vi "Init.vi"(6 "Column Definitions":T9[](array[typedef]) {"MinWidth" min=2 step=1; "AutoSizeMode" items=["None"=1, "ColumnHeader"=2, "AllCellsExceptHeader"=4, "AllCells"=6, "DisplayedCellsExceptHeader"=8, "DisplayedCells"=10, "Fill"=16]; "FillWeight" min=1 max=100}, 7 "Menu Items":string[](array[string])=["Add", "Remove", "Edit"], 8 "error in (no error)":errorcluster, 9 "Node object refs":T1, 10 "Event References":T2, 11 "Multi Column Listbox in":refnum<class "Multi Column Listbox.lvclass">) -> (0 "error out":errorcluster, 2 "Table Events":T13, 3 "Multi Column Listbox out":refnum<class "Multi Column Listbox.lvclass">)   [LabVIEW 2013, in "Table Manager.lvlib" / "Multi Column Listbox.lvclass"]
doc: "This VIs creates the Column Objects that the table will use based on the configuration recived, and register the events the table will use. Also creates the evetns that will be used by the table"
uses:
  Multi Column Listbox.lvclass
  Table Manager/Table Events.ctl
  Table Manager/Menu Select.ctl
  Column/Column Descriptor.ctl
  Column/Column.lvclass
  Column/Column Type.ctl
  <vilib>/NI/Tag Bus/tag/Data Type.ctl
  Table Manager/Call Back Ref Type Def.ctl
  Configuration Editor/Classes/Engine Parent/Engine Parent Editor Node.lvclass
  Configuration Editor/Classes/Module editor node/module editor node.lvclass
  Table Manager/references.ctl
  <vilib>/NI/Configuration Framework/Node/StopEvent.ctl
  <vilib>/NI/Configuration Framework/Node/RefreshUIEvent.ctl
  <vilib>/NI/Configuration Framework/Node/CacheState.ctl
  <vilib>/NI/Configuration Framework/Node/NodeChangeEvent.ctl
  <vilib>/NI/Configuration Framework/Node/NodeRef.ctl
  <vilib>/NI/Configuration Framework/Node/NISE_CEF_Node.lvclass
  control module/editor node/channel action event.ctl
  control module/editor node/dialog output action.ctl
  <vilib>/NI/Tag Bus Module Framework/channel/TBM channel.lvclass
  <vilib>/NI/Tag Bus/tag/tag descriptor.lvclass
  <vilib>/NI/AMC/Message Queue.ctl
  <vilib>/NI/AMC/Message.ctl
  <vilib>/NI/Tools/Keyed Array/KeyedArray.ctl
  <vilib>/NI/Configuration Framework/Node/UserEventRef.ctl
  <vilib>/NI/Configuration Framework/Controls/EventCluster.ctl
  Table Manager/object ref.ctl
  Line/Line.lvclass
  Table Manager/Table Manager.lvclass/Table Manager.ctl
  Multi Column Listbox.lvclass/Multi Column Listbox.ctl
  String Column/String Column.lvclass
  Column/Column.lvclass/Column.ctl
  Listbox Enum Column/List Box Enum Column.lvclass
  Listbox Enum Column/List Box Enum Column.lvclass/List Box Enum Column.ctl
  Mapping Column/Mapping Column.lvclass
  Mapping Column/Mapping Column.lvclass/Mapping Column.ctl
  Line/Line.lvclass/Line.ctl
  Column/Write Header.vi
  Column/Write Read Only.vi
  Column/Write Call Back VI.vi
  Listbox Enum Column/Write Enum Reference.vi
  Mapping Column/Write Channel suffix.vi
  Column/Write Dependencies List.vi
  Mapping Column/Write Data Type Dependecy.vi
  Mapping Column/Write Name Dependecy.vi
  Table Manager/Write ATM.vi
  Read Listbox.vi
  Line/Write Line UID.vi
  Line/Write Columns.vi
  Table Manager/Write Line.vi
  Table Manager/Write Menu Selection.vi
  Table Manager/Write object refs.vi
  control module/editor node/control module editor.lvclass
  Table Manager/Table Manager.lvclass
  <vilib>/NI/Tools/Keyed Array/Tools_KeyedArray.lvlib
  <vilib>/NI/AMC/AMC.lvlib
  <vilib>/NI/Configuration Framework/NISE_CEF_TreeControl.lvlib
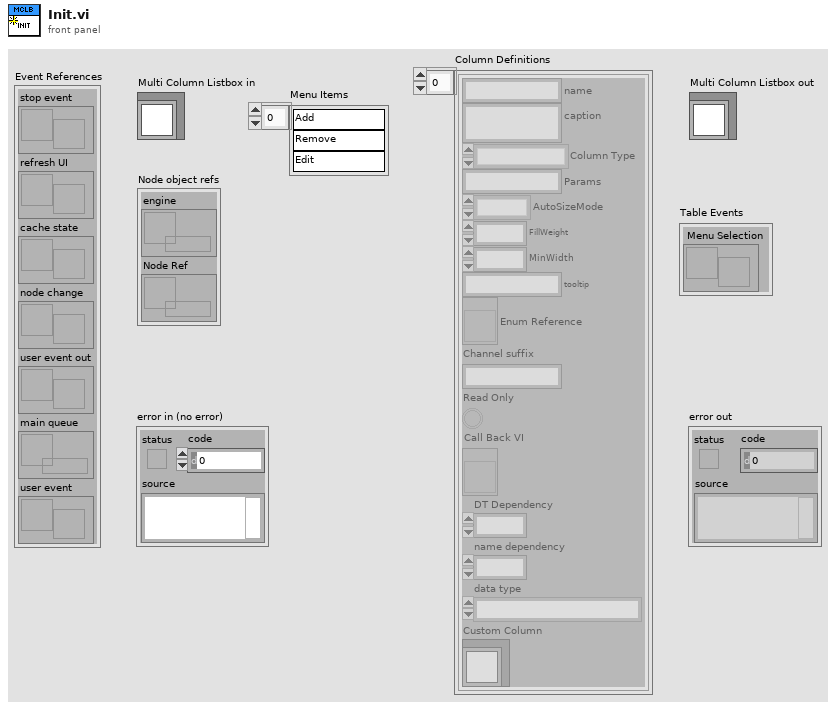
[diagram p1: front panel]
types:
  T1 = typedef "Table Manager.lvlib/Table Manager.lvclass/object ref.ctl" = cluster{"engine":refnum<data-value>, "Node Ref":refnum<data-value>}
  T2 = typedef "Table Manager.lvlib/Table Manager.lvclass/references.ctl" = cluster{"stop event":T3, "refresh UI":T4, "cache state":T5, "node change":T6, "user event out":refnum<user-event>, "main queue":T7, "user event":T8}
  T3 = typedef "NISE_CEF_Node.lvclass/StopEvent.ctl" = refnum<user-event>
  T4 = typedef "NISE_CEF_Node.lvclass/RefreshUIEvent.ctl" = refnum<user-event>
  T5 = typedef "NISE_CEF_Node.lvclass/CacheState.ctl" = refnum<user-event>
  T6 = typedef "NISE_CEF_Node.lvclass/NodeChangeEvent.ctl" = refnum<user-event>
  T7 = typedef "AMC.lvlib/Message Queue.ctl" = refnum<queue>
  T8 = typedef "NISE_CEF_Node.lvclass/UserEventRef.ctl" = refnum<user-event>
  T9 = typedef "Table Manager.lvlib/Column.lvclass/Column Descriptor.ctl" = cluster{"name":string, "caption":string, "Column Type":T10, "Params":string, "AutoSizeMode":i32, "FillWeight":sgl, "MinWidth":u32, "tooltip":string, "Enum Reference":refnum<vi>, "Channel suffix":string, "Read Only":bool, "Call Back VI":T11, "DT Dependency":i32, "name dependency":i32, "data type":T12, "Custom Column":refnum<class "Column.lvclass">}
  T10 = typedef "Table Manager.lvlib/Column.lvclass/Column Type.ctl" = enum16{"String", "Mapping", "Enum", "Custom"}
  T11 = typedef "Table Manager.lvlib/Table Manager.lvclass/Call Back Ref Type Def.ctl" = refnum<vi>
  T12 = typedef "tag bus.lvlib/tag descriptor.lvclass/Data Type.ctl" = enum16{"Double", "Single", "I64", "I32", "I16", "I8", "U64", "U32", "U16", "U8", "Boolean", "String", "Array of Double", "Array of Single", "Array of I64", "Array of I32", "Array of I16", "Array of I8", "Array of U64", "Array of U32", "Array of U16", "Array of U8", "Array of Boolean", "Array of String"}
  T13 = typedef "Table Manager.lvlib/Table Manager.lvclass/Table Events.ctl" = cluster{"Menu Selection":refnum<user-event>}
  T14 = typedef "Table Manager.lvlib/Table Manager.lvclass/Menu Select.ctl" = cluster{"Line Name":string, "Selected Value":string, "Row":i32, "Column":i32, "Table Index":i32}
  T15 = typedef "control module editor.lvclass/channel action event.ctl" = cluster{"action":T16, "channel":refnum<class "TBM channel.lvclass">, "selected tag":refnum<class "tag descriptor.lvclass">}
  T16 = typedef "control module editor.lvclass/dialog output action.ctl" = enum16{"Tag Created", "Tag Selected", "Set Default", "disconnect"}
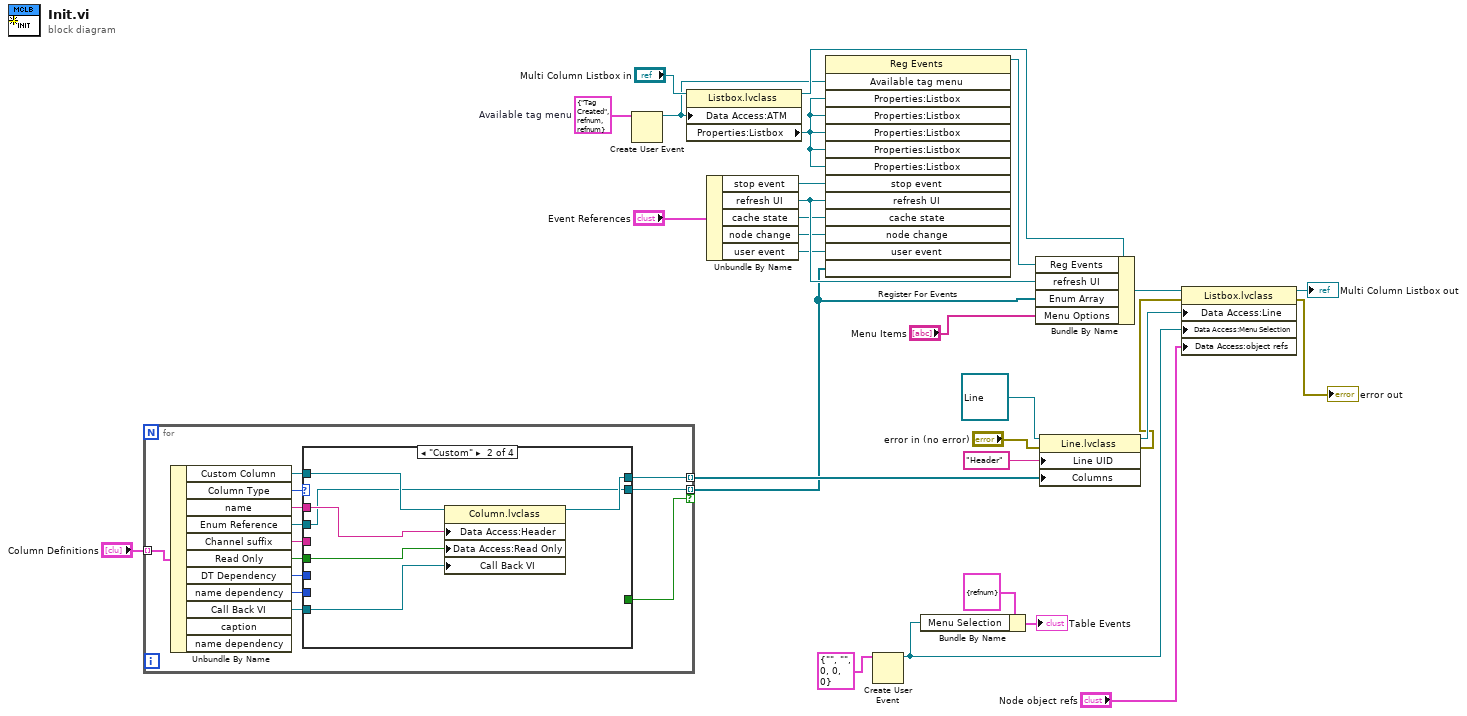
[diagram p0: block diagram]
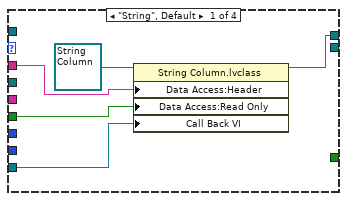
[diagram p2: hidden frame]
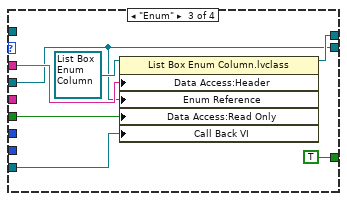
[diagram p3: hidden frame]
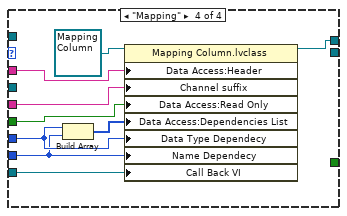
[diagram p4: hidden frame]
diagram:
  w20 = T15 {"action"=enum."Tag Created", "channel"=refnum, "selected tag"=refnum}  # Available tag menu
  n1 = for {
    tunnel: "Column Definitions" -> [w42] mode=indexing
    tunnel: [w40] -> w26 mode=indexing
    tunnel: [w36] -> w11 mode=indexing if=w35
    n2 = Unbundle By Name(w42) -> ("Custom Column"=w30:refnum<class "Column.lvclass">, "Column Type"=w41:T10, "name"=w39:string, "Enum Reference"=w38:refnum<vi>, "Channel suffix"=w37:string, "Read Only"=w34:bool, "DT Dependency"=w33:i32, "name dependency"=w32:i32, "Call Back VI"=w31:T11)  [unwired: 2 out]
    n3 = case shown="\"Custom\"" w41 {
      tunnel: [w45 w52 w59 w68] -> w40
      tunnel: w39 -> [w46 w53 w58 w67]
      tunnel: w38 -> [_ w48 w57 _]
      tunnel: w37 -> [_ _ _ w66]
      tunnel: [_ w48 w57 _] -> w36
      tunnel: [_ _ TRUE _] -> w35
      tunnel: w34 -> [w44 w51 w55 w65]
      tunnel: w33 -> [_ _ _ w63]
      tunnel: w32 -> [_ _ _ w62]
      tunnel: w31 -> [w43 w50 w54 w61]
      tunnel: w30 -> [_ w49 _ _]
      frame "String", Default {
        n4 = property class="String Column.lvclass"(reference=refnum<class "String Column.lvclass"> refnum ("Table Manager.lvlib:String Column.lvclass"), "Data Access:Header"=w46, "Data Access:Read Only"=w44, "Call Back VI"=w43) -> (reference out=w45:refnum<class "String Column.lvclass">)  [unwired: 1 in, 1 out]
      }
      frame "Custom" {
        n5 = property class="Column.lvclass"(reference=w49, "Data Access:Header"=w53, "Data Access:Read Only"=w51, "Call Back VI"=w50) -> (reference out=w52:refnum<class "Column.lvclass">)  [unwired: 1 in, 1 out]
      }
      frame "Enum" {
        n6 = property class="List Box Enum Column.lvclass"(reference=refnum<class "List Box Enum Column.lvclass"> refnum ("Table Manager.lvlib:List Box Enum Column.lvclass"), "Data Access:Header"=w58, "Enum Reference"=w57, "Data Access:Read Only"=w55, "Call Back VI"=w54) -> (reference out=w59:refnum<class "List Box Enum Column.lvclass">)  [unwired: 1 in, 1 out]
      }
      frame "Mapping" {
        n7 = Build Array(w63, w62) -> (w64:i32[])
        n8 = property class="Mapping Column.lvclass"(reference=refnum<class "Mapping Column.lvclass"> refnum ("Table Manager.lvlib:Tag Channel Column.lvclass"), "Data Access:Header"=w67, "Channel suffix"=w66, "Data Access:Read Only"=w65, "Data Access:Dependencies List"=w64, "Data Type Dependecy"=w63, "Name Dependecy"=w62, "Call Back VI"=w61) -> (reference out=w68:refnum<class "Mapping Column.lvclass">)  [unwired: 1 in, 1 out]
      }
    }
  }
  n9 = Create User Event(user event datatype=w20) -> (user event=w19:refnum<user-event>)  [unwired: 1 in, 1 out]
  n10 = property class="Listbox.lvclass"(reference="Multi Column Listbox in", "Data Access:ATM"=w19) -> (reference out=w22:refnum<class "Multi Column Listbox.lvclass">, "Properties:Listbox"=w10:refnum<vi>)  [unwired: 1 in, 1 out]
  n11 = Unbundle By Name("Event References") -> ("stop event"=w17:T3, "refresh UI"=w16:T4, "cache state"=w15:T5, "node change"=w14:T6, "user event"=w13:T8)
  n12 = register-events(w19, w10, w10, w10, w10, w10, w17, w16, w15, w14, w13, w11) -> (reference out=w9:refnum<event-registration>)  [unwired: 2 in, 1 out]
  n13 = Create User Event(user event datatype=T14 {"Line Name"="", "Selected Value"="", "Row"=0, "Column"=0, "Table Index"=0} ("Menu Selection")) -> (user event=w4:refnum<user-event>)  [unwired: 1 in, 1 out]
  n14 = Bundle By Name(cluster=T13 {"Menu Selection"=refnum} ("Table Events"), "Menu Selection"=w4) -> (→"Table Events":T13)
  n15 = Bundle By Name(cluster=w22, "Reg Events"=w9, "refresh UI"=w16, "Enum Array"=w11, "Menu Options"="Menu Items") -> (w21:refnum<class "Multi Column Listbox.lvclass">)
  n16 = property class="Line.lvclass"(reference=refnum<class "Line.lvclass"> refnum ("Table Manager.lvlib:Line.lvclass"), error in="error in (no error)", "Line UID"="Header", "Columns"=w26) -> (reference out=w24:refnum<class "Line.lvclass">, error out=w3:errorcluster)
  n17 = property class="Listbox.lvclass"(reference=w21, error in=w3, "Data Access:Line"=w24, "Data Access:Menu Selection"=w4, "Data Access:object refs"="Node object refs") -> (reference out=→"Multi Column Listbox out":refnum<class "Multi Column Listbox.lvclass">, error out=→"error out":errorcluster)
